vi "Voltage and Current Ring Chooser.vi"(8 "error in (no error)":errorcluster, 11 "Tektronix PA1000 in":refnum<class "Tektronix PA1000.lvclass">) -> (0 "error out":errorcluster, 1 "Current Strings And Values []":T1, 2 "Voltage Strings And Values []":T1, 3 "Tektronix PA1000 out":refnum<class "Tektronix PA1000.lvclass">, 4 "Wiring Strings And Values []":T1)   [LabVIEW 2013, in "Universal Power Meter.lvlib" / "Tektronix PA1000.lvlib" / "Tektronix PA1000.lvclass"]
uses:
  Tektronix PA1000.lvclass
  <vilib>/Utility/miscctls.llb/LVStringsAndValuesArrayTypeDef_U16.ctl
  Universal Power Meter class/Universal Power Meter.lvclass
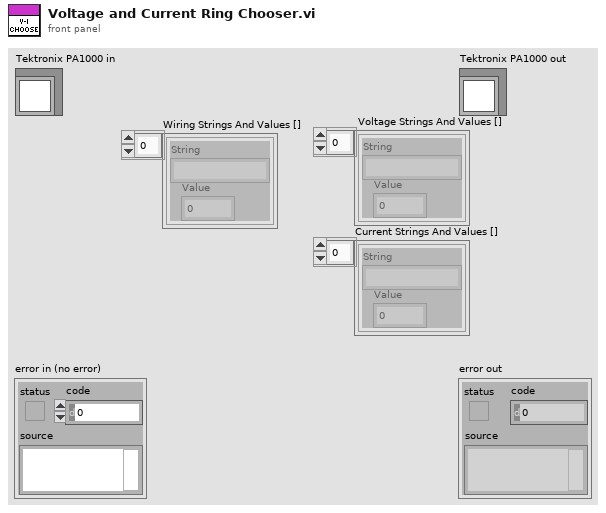
[diagram p1: front panel]
types:
  T1 = typedef "LVStringsAndValuesArrayTypeDef_U16.ctl" = cluster{"String":string, "Value":u16}[]
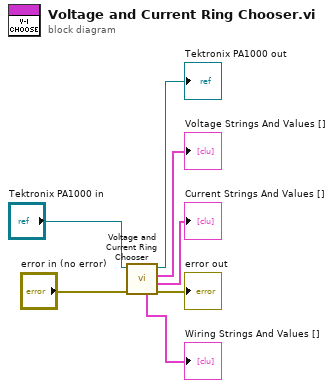
[diagram p0: block diagram]
diagram:
  n1 = call-parent "Voltage and Current Ring Chooser.vi"("error in (no error)"="error in (no error)", "Universal Power Meter in"="Tektronix PA1000 in") -> ("error out"=→"error out":errorcluster, "Current Strings And Values []"=→"Current Strings And Values []":T1, "Voltage Strings And Values []"=→"Voltage Strings And Values []":T1, "Universal Power Meter out"=→"Tektronix PA1000 out":refnum<class "Tektronix PA1000.lvclass">, "Wiring Strings And Values []"=→"Wiring Strings And Values []":T1)  [unwired: 5 in]
